vi "log analysis_gps.vi"() -> ()   [LabVIEW 2019] (continued)
 "DUALANTENNAHEADINGA,USB3,0,50.0,FINESTEERING,2107,283656.700,02000000,d426,15824;INSUFFICIENT_OBS,NONE,-1.000000000,0.000000000,0.000000000,0.0,0.000000000,0.000000000,\"631T\",13,4,4,3,04,00,20,03*b691e1de\n\t", "DUALANTENNAHEADINGA,USB3,0,48.0,FINESTEERING,2107,283657.200,02000000,d426,15824;INSUFFICIENT_OBS,NONE,-1.000000000,0.000000000,0.000000000,0.0,0.000000000,0.000000000,\"631T\",13,4,4,3,04,00,20,02*3e465e4d\n\t", "DUALANTENNAHEADINGA,USB3,0,48.0,FINESTEERING,2107,283657.700,02000000,d426,15824;INSUFFICIENT_OBS,NONE,-1.000000000,0.000000000,0.000000000,0.0,0.000000000,0.000000000,\"631T\",13,4,4,3,04,00,20,02*e9554f14\n\t", "INSPVAXA,USB3,0,51.0,FINESTEERING,2107,283658.200,02000000,471d,15824;INS_ALIGNMENT_COMPLETE,INS_RTKFIXED,37.37126197205,126.72203987070,7.8924,22.3000,0.0140,-0.2985,0.0088,-0.407757942,-1.836378522,264.980716512,0.4370,0.2959,0.5779,0.1123,0.0925,0.0785,0.0961,0.1008,5.1265,0f000001,0*c213c735\n\t", "DUALANTENNAHEADINGA,USB3,0,51.0,FINESTEERING,2107,283658.700,02000000,d426,15824;INSUFFICIENT_OBS,NONE,-1.000000000,0.000000000,0.000000000,0.0,0.000000000,0.000000000,\"631T\",14,4,4,3,04,00,20,02*806fba7a\n\t", "DUALANTENNAHEADINGA,USB3,0,45.5,FINESTEERING,2107,283659.200,02000000,d426,15824;INSUFFICIENT_OBS,NONE,-1.000000000,0.000000000,0.000000000,0.0,0.000000000,0.000000000,\"631T\",13,4,4,3,04,00,20,02*be5dbd8b\n\t", "INSPVAXA,USB3,0,45.5,FINESTEERING,2107,283659.700,02000000,471d,15824;INS_ALIGNMENT_COMPLETE,INS_RTKFIXED,37.37126196302,126.72203492233,7.8846,22.3000,0.0219,-0.3038,0.0154,-0.352814130,-1.840091471,265.280226018,0.4363,0.2959,0.5779,0.1123,0.0925,0.0785,0.0961,0.1008,5.1280,0f000001,0*f5025ff3\n\t", "DUALANTENNAHEADINGA,USB3,0,48.5,FINESTEERING,2107,283660.200,02000000,d426,15824;INSUFFICIENT_OBS,NONE,-1.000000000,0.000000000,0.000000000,0.0,0.000000000,0.000000000,\"631T\",14,4,4,3,04,00,20,02*21adfb59\n\t", "DUALANTENNAHEADINGA,USB3,0,48.5,FINESTEERING,2107,283660.700,02000000,d426,15824;INSUFFICIENT_OBS,NONE,-1.000000000,0.000000000,0.000000000,0.0,0.000000000,0.000000000,\"631T\",15,4,4,3,04,00,20,03*565b5ace\n\t", "INSPVAXA,USB3,0,49.5,FINESTEERING,2107,283661.200,02000000,471d,15824;INS_ALIGNMENT_COMPLETE,INS_RTKFIXED,37.37126187130,126.72202999654,7.8827,22.3000,0.0166,-0.2769,0.0144,-0.534535443,-1.728487239,265.001971487,0.4359,0.2961,0.5778,0.1123,0.0926,0.0785,0.0961,0.1008,5.1311,0f000001,0*51cc925f\n\t", "DUALANTENNAHEADINGA,USB3,0,49.5,FINESTEERING,2107,283661.700,02000000,d426,15824;INSUFFICIENT_OBS,NONE,-1.000000000,0.000000000,0.000000000,0.0,0.000000000,0.000000000,\"631T\",12,4,4,3,04,00,20,03*15f903f8\n\t", "DUALANTENNAHEADINGA,USB3,0,48.0,FINESTEERING,2107,283662.200,02000000,d426,15824;INSUFFICIENT_OBS,NONE,-1.000000000,0.000000000,0.000000000,0.0,0.000000000,0.000000000,\"631T\",12,4,4,3,04,00,20,03*45bc2fa2\n\t", "INSPVAXA,USB3,0,48.0,FINESTEERING,2107,283662.700,02000000,471d,15824;INS_ALIGNMENT_COMPLETE,INS_RTKFIXED,37.37126171572,126.72202522799,7.8823,22.3000,-0.0067,-0.2635,0.0136,-1.179961552,0.094212856,265.044425368,0.4362,0.2961,0.5779,0.1131,0.0926,0.0785,0.0961,0.1008,5.1327,0f000001,0*9a1b8d6f\n\t", "DUALANTENNAHEADINGA,USB3,0,49.0,FINESTEERING,2107,283663.200,02000000,d426,15824;INSUFFICIENT_OBS,NONE,-1.000000000,0.000000000,0.000000000,0.0,0.000000000,0.000000000,\"631T\",12,4,4,3,04,00,20,03*4c20fddf\n\t", "DUALANTENNAHEADINGA,USB3,0,49.0,FINESTEERING,2107,283663.700,02000000,d426,15824;INSUFFICIENT_OBS,NONE,-1.000000000,0.000000000,0.000000000,0.0,0.000000000,0.000000000,\"631T\",13,4,4,3,04,00,20,03*4cd16cde\n\t", "DUALANTENNAHEADINGA,USB3,0,53.0,FINESTEERING,2107,283664.200,02000000,d426,15824;INSUFFICIENT_OBS,NONE,-1.000000000,0.000000000,0.000000000,0.0,0.000000000,0.000000000,\"631T\",14,4,4,3,04,00,20,02*f110e9d9\n\t", "DUALANTENNAHEADINGA,USB3,0,53.0,FINESTEERING,2107,283664.700,02000000,d426,15824;INSUFFICIENT_OBS,NONE,-1.000000000,0.000000000,0.000000000,0.0,0.000000000,0.000000000,\"631T\",15,4,4,3,04,00,20,02*f1e178d8\n\t", "DUALANTENNAHEADINGA,USB3,0,50.0,FINESTEERING,2107,283665.200,02000000,d426,15824;INSUFFICIENT_OBS,NONE,-1.000000000,0.000000000,0.000000000,0.0,0.000000000,0.000000000,\"631T\",13,4,4,3,04,00,20,03*0d3c2d31\n\t", "DUALANTENNAHEADINGA,USB3,0,50.0,FINESTEERING,2107,283665.700,02000000,d426,15824;INSUFFICIENT_OBS,NONE,-1.000000000,0.000000000,0.000000000,0.0,0.000000000,0.000000000,\"631T\",12,4,4,3,04,00,20,02*7aca8ca6\n\t", "DUALANTENNAHEADINGA,USB3,0,49.5,FINESTEERING,2107,283666.200,02000000,d426,15824;INSUFFICIENT_OBS,NONE,-1.000000000,0.000000000,0.000000000,0.0,0.000000000,0.000000000,\"631T\",12,4,4,3,04,00,20,03*18930aef\n\t", "DUALANTENNAHEADINGA,USB3,0,51.0,FINESTEERING,2107,283667.200,02000000,d426,15824;INSUFFICIENT_OBS,NONE,-1.000000000,0.000000000,0.000000000,0.0,0.000000000,0.000000000,\"631T\",14,4,4,3,04,00,20,03*f8f6796c\n\t", "DUALANTENNAHEADINGA,USB3,0,51.0,FINESTEERING,2107,283667.700,02000000,d426,15824;INSUFFICIENT_OBS,NONE,-1.000000000,0.000000000,0.000000000,0.0,0.000000000,0.000000000,\"631T\",14,4,4,3,04,00,20,02*58e258a3\n\t", "DUALANTENNAHEADINGA,USB3,0,51.5,FINESTEERING,2107,283668.200,02000000,d426,15824;INSUFFICIENT_OBS,NONE,-1.000000000,0.000000000,0.000000000,0.0,0.000000000,0.000000000,\"631T\",13,4,4,3,04,00,20,03*e5e926ef\n\t", "DUALANTENNAHEADINGA,USB3,0,51.5,FINESTEERING,2107,283668.700,02000000,d426,15824;INSUFFICIENT_OBS,NONE,-1.000000000,0.000000000,0.000000000,0.0,0.000000000,0.000000000,\"631T\",12,4,4,3,04,00,20,03*e518b7ee\n\t", "DUALANTENNAHEADINGA,USB3,0,49.0,FINESTEERING,2107,283669.200,02000000,d426,15824;INSUFFICIENT_OBS,NONE,-1.000000000,0.000000000,0.000000000,0.0,0.000000000,0.000000000,\"631T\",12,4,4,3,04,00,20,03*4fb2de27\n\t", "DUALANTENNAHEADINGA,USB3,0,49.0,FINESTEERING,2107,283669.700,02000000,d426,15824;INSUFFICIENT_OBS,NONE,-1.000000000,0.000000000,0.000000000,0.0,0.000000000,0.000000000,\"631T\",12,4,4,3,04,00,20,02*efa6ffe8\n\t", "DUALANTENNAHEADINGA,USB3,0,50.0,FINESTEERING,2107,283670.200,02000000,d426,15824;INSUFFICIENT_OBS,NONE,-1.000000000,0.000000000,0.000000000,0.0,0.000000000,0.000000000,\"631T\",12,4,4,3,04,00,20,03*24750ee1\n\t", "DUALANTENNAHEADINGA,USB3,0,50.0,FINESTEERING,2107,283670.700,02000000,d426,15824;INSUFFICIENT_OBS,NONE,-1.000000000,0.000000000,0.000000000,0.0,0.000000000,0.000000000,\"631T\",13,4,4,3,04,00,20,03*24849fe0\n\t", "DUALANTENNAHEADINGA,USB3,0,50.0,FINESTEERING,2107,283671.200,02000000,d426,15824;INSUFFICIENT_OBS,NONE,-1.000000000,0.000000000,0.000000000,0.0,0.000000000,0.000000000,\"631T\",13,4,4,3,04,00,20,02*e948baf6\n\t", "DUALANTENNAHEADINGA,USB3,0,50.0,FINESTEERING,2107,283671.700,02000000,d426,15824;INSUFFICIENT_OBS,NONE,-1.000000000,0.000000000,0.000000000,0.0,0.000000000,0.000000000,\"631T\",12,4,4,3,04,00,20,02*e9b92bf7\n\t", "DUALANTENNAHEADINGA,USB3,0,47.5,FINESTEERING,2107,283672.200,02000000,d426,15824;INSUFFICIENT_OBS,NONE,-1.000000000,0.000000000,0.000000000,0.0,0.000000000,0.000000000,\"631T\",13,4,4,3,04,00,20,03*4a2d65dd\n\t", "DUALANTENNAHEADINGA,USB3,0,47.5,FINESTEERING,2107,283672.700,02000000,d426,15824;INSUFFICIENT_OBS,NONE,-1.000000000,0.000000000,0.000000000,0.0,0.000000000,0.000000000,\"631T\",11,4,4,3,04,00,20,03*e98a7275\n\t", "DUALANTENNAHEADINGA,USB3,0,49.0,FINESTEERING,2107,283673.200,02000000,d426,15824;INSUFFICIENT_OBS,NONE,-1.000000000,0.000000000,0.000000000,0.0,0.000000000,0.000000000,\"631T\",12,4,4,3,04,00,20,02*c4457f3d\n\t", "DUALANTENNAHEADINGA,USB3,0,49.0,FINESTEERING,2107,283673.700,02000000,d426,15824;INSUFFICIENT_OBS,NONE,-1.000000000,0.000000000,0.000000000,0.0,0.000000000,0.000000000,\"631T\",13,4,4,3,04,00,20,03*b3b3deaa\n\t", "DUALANTENNAHEADINGA,USB3,0,50.0,FINESTEERING,2107,283674.200,02000000,d426,15824;INSUFFICIENT_OBS,NONE,-1.000000000,0.000000000,0.000000000,0.0,0.000000000,0.000000000,\"631T\",13,4,4,3,04,00,20,03*9f869b9c\n\t", "INSPVAXA,USB3,0,50.0,FINESTEERING,2107,283674.750,02000000,471d,15824;INS_ALIGNMENT_COMPLETE,INS_RTKFIXED,37.37126252882,126.72198672229,7.9795,22.3000,-0.0186,-0.2998,0.0327,-1.236759140,0.298585225,263.242315357,0.4398,0.2975,0.5789,0.1131,0.0929,0.0786,0.0960,0.1008,5.0828,0f000001,0*30bc741b\n\t", "DUALANTENNAHEADINGA,USB3,0,47.5,FINESTEERING,2107,283675.200,02000000,d426,15824;INSUFFICIENT_OBS,NONE,-1.000000000,0.000000000,0.000000000,0.0,0.000000000,0.000000000,\"631T\",12,4,4,3,04,00,20,02*30b1cd5d\n\t", "DUALANTENNAHEADINGA,USB3,0,47.5,FINESTEERING,2107,283675.700,02000000,d426,15824;INSUFFICIENT_OBS,NONE,-1.000000000,0.000000000,0.000000000,0.0,0.000000000,0.000000000,\"631T\",13,4,4,3,04,00,20,03*47476cca\n\t", "DUALANTENNAHEADINGA,USB3,0,50.0,FINESTEERING,2107,283676.200,02000000,d426,15824;INSUFFICIENT_OBS,NONE,-1.000000000,0.000000000,0.000000000,0.0,0.000000000,0.000000000,\"631T\",13,4,4,3,04,00,20,02*3331a2b8\n\t", "INSPVAXA,USB3,0,50.0,FINESTEERING,2107,283676.750,02000000,471d,15824;INS_ALIGNMENT_COMPLETE,INS_RTKFIXED,37.37126202802,126.72198037867,7.9931,22.3000,-0.0270,-0.2983,0.0289,-1.276938431,0.174085147,258.154591337,0.4371,0.2976,0.5788,0.1128,0.0927,0.0785,0.0959,0.1007,5.0828,0f000001,0*1eb9a34f\n\t", "INSPVAXA,USB3,0,47.5,FINESTEERING,2107,283677.250,02000000,471d,15824;INS_ALIGNMENT_COMPLETE,INS_RTKFIXED,37.37126184306,126.72197878066,7.9954,22.3000,-0.0249,-0.2800,0.0095,-1.329008924,0.068233484,257.455385518,0.4363,0.2976,0.5789,0.1128,0.0926,0.0785,0.0959,0.1006,5.0823,0f000001,0*a0488656\n\t", "INSPVAXA,USB3,0,44.5,FINESTEERING,2107,283678.750,02000000,471d,15824;INS_ALIGNMENT_COMPLETE,INS_RTKFIXED,37.37126126052,126.72197417876,8.0025,22.3000,-0.0388,-0.3139,0.0075,-1.341441151,0.143163163,255.994609032,0.4352,0.2975,0.5790,0.1123,0.0928,0.0785,0.0959,0.1006,5.0816,0f000001,0*2dcb75ae\n\t", "INSPVAXA,USB3,0,50.0,FINESTEERING,2107,283679.250,02000000,471d,15824;INS_ALIGNMENT_COMPLETE,INS_RTKFIXED,37.37126102386,126.72197256335,8.0029,22.3000,-0.0378,-0.3051,0.0239,-1.252291621,0.317106039,255.710782643,0.4355,0.2977,0.5792,0.1125,0.0927,0.0786,0.0959,0.1006,5.0819,0f000001,0*497f861f\n\t", "DUALANTENNAHEADINGA,USB3,0,50.0,FINESTEERING,2107,283679.700,02000000,d426,15824;INSUFFICIENT_OBS,NONE,-1.000000000,0.000000000,0.000000000,0.0,0.000000000,0.000000000,\"631T\",13,4,4,3,04,00,20,03*917eb173\n\t", "INSPVAXA,USB3,0,49.5,FINESTEERING,2107,283680.250,02000000,471d,15824;INS_ALIGNMENT_COMPLETE,INS_RTKFIXED,37.37126052998,126.72196935056,8.0055,22.3000,-0.0369,-0.2979,0.0271,-1.221523222,0.248269535,255.390291305,0.4350,0.2975,0.5791,0.1126,0.0927,0.0786,0.0959,0.1006,5.0824,0f000001,0*4c9222e8\n\t", "INSPVAXA,USB3,0,49.5,FINESTEERING,2107,283680.750,02000000,471d,15824;INS_ALIGNMENT_COMPLETE,INS_RTKFIXED,37.37126029067,126.72196774054,8.0075,22.3000,-0.0484,-0.2930,0.0156,-1.123777574,0.215686141,255.306454627,0.4350,0.2975,0.5791,0.1126,0.0927,0.0786,0.0959,0.1006,5.0824,0f000001,0*b1d08eab\n\t", "DUALANTENNAHEADINGA,USB3,0,47.5,FINESTEERING,2107,283681.200,02000000,d426,15824;INSUFFICIENT_OBS,NONE,-1.000000000,0.000000000,0.000000000,0.0,0.000000000,0.000000000,\"631T\",13,4,4,3,04,00,20,02*8c2dc70b\n\t", "DUALANTENNAHEADINGA,USB3,0,47.5,FINESTEERING,2107,283681.700,02000000,d426,15824;INSUFFICIENT_OBS,NONE,-1.000000000,0.000000000,0.000000000,0.0,0.000000000,0.000000000,\"631T\",13,4,4,3,04,00,20,03*2c39e6c4\n\t", "DUALANTENNAHEADINGA,USB3,0,53.0,FINESTEERING,2107,283682.200,02000000,d426,15824;INSUFFICIENT_OBS,NONE,-1.000000000,0.000000000,0.000000000,0.0,0.000000000,0.000000000,\"631T\",13,4,4,3,04,00,20,02*f482535a\n\t", "INSPVAXA,USB3,0,53.0,FINESTEERING,2107,283682.750,02000000,471d,15824;INS_ALIGNMENT_COMPLETE,INS_RTKFIXED,37.37125926494,126.72196137618,8.0142,22.3000,-0.0531,-0.2940,0.0193,-1.467222683,0.192661373,255.088191975,0.4346,0.2973,0.5792,0.1126,0.0928,0.0786,0.0959,0.1005,5.0834,0f000001,0*e49cbeff\n\t", "DUALANTENNAHEADINGA,USB3,0,51.5,FINESTEERING,2107,283683.200,02000000,d426,15824;INSUFFICIENT_OBS,NONE,-1.000000000,0.000000000,0.000000000,0.0,0.000000000,0.000000000,\"631T\",13,4,4,3,04,00,20,03*73ae2c91\n\t", "INSPVAXA,USB3,0,51.5,FINESTEERING,2107,283683.750,02000000,471d,15824;INS_ALIGNMENT_COMPLETE,INS_RTKFIXED,37.37125874592,126.72195815928,8.0147,22.3000,-0.0440,-0.2967,0.0132,-1.341050050,-0.067435832,254.924614252,0.4345,0.2971,0.5791,0.1126,0.0928,0.0785,0.0959,0.1005,5.0840,0f000001,0*701f89f0\n\t", "DUALANTENNAHEADINGA,USB3,0,52.0,FINESTEERING,2107,283684.200,02000000,d426,15824;INSUFFICIENT_OBS,NONE,-1.000000000,0.000000000,0.000000000,0.0,0.000000000,0.000000000,\"631T\",13,4,4,3,04,00,20,02*27679969\n\t", "INSPVAXA,USB3,0,52.0,FINESTEERING,2107,283684.750,02000000,471d,15824;INS_ALIGNMENT_COMPLETE,INS_RTKFIXED,37.37125823226,126.72195499542,8.0159,22.3000,-0.0425,-0.2912,0.0233,-1.481512417,-0.232627459,254.717814630,0.4345,0.2970,0.5790,0.1126,0.0928,0.0785,0.0959,0.1005,5.0847,0f000001,0*bc004070\n\t", "DUALANTENNAHEADINGA,USB3,0,54.0,FINESTEERING,2107,283685.200,02000000,d426,15824;INSUFFICIENT_OBS,NONE,-1.000000000,0.000000000,0.000000000,0.0,0.000000000,0.000000000,\"631T\",13,4,4,3,04,00,20,03*bf535cbf\n\t", "DUALANTENNAHEADINGA,USB3,0,54.0,FINESTEERING,2107,283685.700,02000000,d426,15824;INSUFFICIENT_OBS,NONE,-1.000000000,0.000000000,0.000000000,0.0,0.000000000,0.000000000,\"631T\",15,4,4,3,04,00,20,03*f59c46f5\n\t", "INSPVAXA,USB3,0,47.0,FINESTEERING,2107,283686.250,02000000,471d,15824;INS_ALIGNMENT_COMPLETE,INS_RTKFIXED,37.37125745168,126.72195028422,8.0177,22.3000,-0.0421,-0.2788,0.0295,-1.327379585,-0.197998940,254.015433265,0.4342,0.2970,0.5788,0.1125,0.0928,0.0785,0.0959,0.1004,5.0859,0f000001,0*059a606c\n\t", "INSPVAXA,USB3,0,47.0,FINESTEERING,2107,283686.750,02000000,471d,15824;INS_ALIGNMENT_COMPLETE,INS_RTKFIXED,37.37125719652,126.72194873669,8.0201,22.3000,-0.0424,-0.2865,0.0311,-1.155721868,-0.143426026,253.623399398,0.4342,0.2970,0.5788,0.1125,0.0928,0.0785,0.0959,0.1004,5.0859,0f000001,0*874a06ff\n\t", "INSPVAXA,USB3,0,48.5,FINESTEERING,2107,283687.250,02000000,471d,15824;INS_ALIGNMENT_COMPLETE,INS_RTKFIXED,37.37125692308,126.72194717786,8.0216,22.3000,-0.0335,-0.2418,0.0315,-1.192319582,-0.154191109,253.231237079,0.4341,0.2971,0.5788,0.1124,0.0928,0.0785,0.0959,0.1004,5.0866,0f000001,0*54818d56\n\t", "INSPVAXA,USB3,0,48.0,FINESTEERING,2107,283688.250,02000000,471d,15824;INS_ALIGNMENT_COMPLETE,INS_RTKFIXED,37.37125642172,126.72194437677,8.0235,22.3000,-0.0500,-0.3046,0.0059,-1.164662178,-0.014385646,252.588332690,0.4343,0.2973,0.5789,0.1124,0.0928,0.0785,0.0959,0.1004,5.0876,0f000001,0*78a62f40\n\t", "INSPVAXA,USB3,0,48.0,FINESTEERING,2107,283688.750,02000000,471d,15824;INS_ALIGNMENT_COMPLETE,INS_RTKFIXED,37.37125610282,126.72194283979,8.0244,22.3000,-0.0543,-0.2923,0.0224,-1.111219856,-0.008949492,252.070206998,0.4343,0.2973,0.5789,0.1124,0.0928,0.0785,0.0959,0.1004,5.0876,0f000001,0*c44a5f5d\n\t", "INSPVAXA,USB3,0,50.0,FINESTEERING,2107,283689.250,02000000,471d,15824;INS_ALIGNMENT_COMPLETE,INS_RTKFIXED,37.37125577091,126.72194129043,8.0250,22.3000,-0.0553,-0.2846,0.0299,-1.126484070,-0.034453614,251.571777713,0.4347,0.2976,0.5789,0.1123,0.0927,0.0785,0.0959,0.1004,5.0890,0f000001,0*4752c184\n\t", "INSPVAXA,USB3,0,50.0,FINESTEERING,2107,283689.750,02000000,471d,15824;INS_ALIGNMENT_COMPLETE,INS_RTKFIXED,37.37125543079,126.72193970784,8.0254,22.3000,-0.0623,-0.2845,0.0344,-1.115085970,-0.181471482,251.113733002,0.4347,0.2976,0.5789,0.1123,0.0927,0.0785,0.0959,0.1004,5.0890,0f000001,0*e6043553\n\t", "INSPVAXA,USB3,0,51.5,FINESTEERING,2107,283690.250,02000000,471d,15824;INS_ALIGNMENT_COMPLETE,INS_RTKFIXED,37.37125508435,126.72193816260,8.0268,22.3000,-0.0829,-0.2745,0.0314,-1.131096634,-0.362526816,250.672431743,0.4348,0.2977,0.5789,0.1123,0.0927,0.0785,0.0959,0.1004,5.0905,0f000001,0*0f3c6f4d\n\t", "INSPVAXA,USB3,0,51.5,FINESTEERING,2107,283690.750,02000000,471d,15824;INS_ALIGNMENT_COMPLETE,INS_RTKFIXED,37.37125472381,126.72193660268,8.0270,22.3000,-0.0761,-0.2693,0.0189,-1.124428932,-0.555258111,250.148936400,0.4348,0.2977,0.5789,0.1123,0.0927,0.0785,0.0959,0.1004,5.0905,0f000001,0*bccc2e0c\n\t", "INSPVAXA,USB3,0,51.0,FINESTEERING,2107,283691.250,02000000,471d,15824;INS_ALIGNMENT_COMPLETE,INS_RTKFIXED,37.37125435874,126.72193505456,8.0263,22.3000,-0.0670,-0.2696,0.0092,-1.064456242,-0.547416950,249.737681282,0.4347,0.2977,0.5789,0.1123,0.0927,0.0785,0.0959,0.1004,5.0921,0f000001,0*f2a7f55d\n\t", "INSPVAXA,USB3,0,51.0,FINESTEERING,2107,283691.750,02000000,471d,15824;INS_ALIGNMENT_COMPLETE,INS_RTKFIXED,37.37125397017,126.72193349362,8.0255,22.3000,-0.0691,-0.2936,0.0158,-1.034003666,-0.605283129,249.246949956,0.4347,0.2977,0.5789,0.1123,0.0927,0.0785,0.0959,0.1004,5.0921,0f000001,0*27b79f83\n\t", "INSPVAXA,USB3,0,52.0,FINESTEERING,2107,283692.250,02000000,471d,15824;INS_ALIGNMENT_COMPLETE,INS_RTKFIXED,37.37125358988,126.72193199872,8.0234,22.3000,-0.0664,-0.2884,0.0105,-1.029506848,-0.448748893,248.703805210,0.4344,0.2976,0.5789,0.1123,0.0927,0.0785,0.0960,0.1004,5.0936,0f000001,0*b0abd4b9\n\t", "INSPVAXA,USB3,0,52.0,FINESTEERING,2107,283692.750,02000000,471d,15824;INS_ALIGNMENT_COMPLETE,INS_RTKFIXED,37.37125319556,126.72193048668,8.0218,22.3000,-0.0721,-0.2829,0.0182,-0.873709041,-0.554913446,248.258505340,0.4344,0.2976,0.5789,0.1123,0.0927,0.0785,0.0960,0.1004,5.0936,0f000001,0*33541c24\n\t", "INSPVAXA,USB3,0,52.0,FINESTEERING,2107,283693.250,02000000,471d,15824;INS_ALIGNMENT_COMPLETE,INS_RTKFIXED,37.37125278430,126.72192895782,8.0198,22.3000,-0.0808,-0.2833,0.0124,-0.750595920,-0.512604817,247.887825209,0.4345,0.2977,0.5790,0.1123,0.0927,0.0785,0.0960,0.1005,5.0951,0f000001,0*33503232\n\t", "INSPVAXA,USB3,0,52.0,FINESTEERING,2107,283693.750,02000000,471d,15824;INS_ALIGNMENT_COMPLETE,INS_RTKFIXED,37.37125237385,126.72192745643,8.0181,22.3000,-0.0699,-0.2766,0.0107,-0.708441706,-0.569028922,247.469165126,0.4345,0.2977,0.5790,0.1123,0.0927,0.0785,0.0960,0.1005,5.0951,0f000001,0*b12f53f8\n\t", "INSPVAXA,USB3,0,51.5,FINESTEERING,2107,283694.250,02000000,471d,15824;INS_ALIGNMENT_COMPLETE,INS_RTKFIXED,37.37125195619,126.72192597903,8.0151,22.3000,-0.0814,-0.2811,0.0110,-0.711365496,-0.463120250,247.118464084,0.4343,0.2979,0.5790,0.1123,0.0927,0.0785,0.0960,0.1005,5.0966,0f000001,0*fc596ab1\n\t", "INSPVAXA,USB3,0,51.5,FINESTEERING,2107,283694.750,02000000,471d,15824;INS_ALIGNMENT_COMPLETE,INS_RTKFIXED,37.37125151893,126.72192448231,8.0119,22.3000,-0.0800,-0.2663,0.0091,-0.771660159,-0.376939407,246.768281160,0.4343,0.2979,0.5790,0.1123,0.0927,0.0785,0.0960,0.1005,5.0966,0f000001,0*6d22b1be\n\t", "INSPVAXA,USB3,0,48.0,FINESTEERING,2107,283695.250,02000000,471d,15824;INS_ALIGNMENT_COMPLETE,INS_RTKFIXED,37.37125106123,126.72192297885,8.0100,22.3000,-0.0761,-0.2505,0.0231,-0.897100380,-0.291610583,246.370264659,0.4345,0.2982,0.5790,0.1123,0.0927,0.0785,0.0960,0.1005,5.0981,0f000001,0*3984aa9f\n\t", "INSPVAXA,USB3,0,48.0,FINESTEERING,2107,283695.750,02000000,471d,15824;INS_ALIGNMENT_COMPLETE,INS_RTKFIXED,37.37125059397,126.72192150260,8.0095,22.3000,-0.0806,-0.2555,0.0180,-1.082975458,-0.280956917,246.024954508,0.4345,0.2982,0.5790,0.1123,0.0927,0.0785,0.0960,0.1005,5.0981,0f000001,0*61086754\n\t", "INSPVAXA,USB3,0,48.5,FINESTEERING,2107,283696.250,02000000,471d,15824;INS_ALIGNMENT_COMPLETE,INS_RTKFIXED,37.37125013310,126.72192002149,8.0081,22.3000,-0.0880,-0.2655,0.0330,-1.084281837,-0.279647129,245.685810619,0.4346,0.2982,0.5792,0.1123,0.0927,0.0785,0.0960,0.1005,5.0996,0f000001,0*ddc3e251\n\t", "INSPVAXA,USB3,0,48.5,FINESTEERING,2107,283696.750,02000000,471d,15824;INS_ALIGNMENT_COMPLETE,INS_RTKFIXED,37.37124978634,126.72191884253,8.0066,22.3000,0.0400,0.0236,0.0167,-1.049670935,-0.308268923,245.402478860,0.4346,0.2982,0.5792,0.1123,0.0927,0.0785,0.0960,0.1005,5.0996,0f000001,0*5343d95d\n\t", "INSPVAXA,USB3,0,49.5,FINESTEERING,2107,283697.250,02000000,471d,15824;INS_ALIGNMENT_COMPLETE,INS_RTKFIXED,37.37124936191,126.72191751580,8.0075,22.3000,-0.0790,-0.2224,0.0305,-1.160332211,-0.255386119,245.257033584,0.4348,0.2981,0.5792,0.1123,0.0927,0.0785,0.0960,0.1005,5.1012,0f000001,0*9bb241a9\n\t", "INSPVAXA,USB3,0,49.5,FINESTEERING,2107,283697.750,02000000,471d,15824;INS_ALIGNMENT_COMPLETE,INS_RTKFIXED,37.37124887882,126.72191610954,8.0072,22.3000,-0.0796,-0.2609,0.0250,-1.450872911,-0.189081024,245.072886035,0.4348,0.2981,0.5792,0.1123,0.0927,0.0785,0.0960,0.1005,5.1012,0f000001,0*ca3e42a8\n\t", "INSPVAXA,USB3,0,47.0,FINESTEERING,2107,283698.250,02000000,471d,15824;INS_ALIGNMENT_COMPLETE,INS_RTKFIXED,37.37124839401,126.72191465708,8.0076,22.3000,-0.0773,-0.2590,0.0230,-1.479636169,-0.110505972,244.843169403,0.4347,0.2979,0.5791,0.1126,0.0927,0.0785,0.0960,0.1005,5.1027,0f000001,0*0006d84b\n\t", "INSPVAXA,USB3,0,47.0,FINESTEERING,2107,283698.750,02000000,471d,15824;INS_ALIGNMENT_COMPLETE,INS_RTKFIXED,37.37124790607,126.72191317649,8.0096,22.3000,-0.0919,-0.2605,0.0162,-1.323665543,0.178775756,244.574454938,0.4347,0.2979,0.5791,0.1126,0.0927,0.0785,0.0960,0.1005,5.1027,0f000001,0*97fdd670\n\t", "INSPVAXA,USB3,0,47.5,FINESTEERING,2107,283699.250,02000000,471d,15824;INS_ALIGNMENT_COMPLETE,INS_RTKFIXED,37.37124741280,126.72191168515,8.0116,22.3000,-0.0880,-0.2650,0.0236,-1.277654114,0.173050319,244.335495990,0.4352,0.2978,0.5791,0.1127,0.0927,0.0785,0.0959,0.1005,5.1036,0f000001,0*401d1919\n\t", "INSPVAXA,USB3,0,47.5,FINESTEERING,2107,283699.750,02000000,471d,15824;INS_ALIGNMENT_COMPLETE,INS_RTKFIXED,37.37124691977,126.72191021065,8.0139,22.3000,-0.0941,-0.2573,0.0260,-1.295740084,0.118148751,244.043765881,0.4352,0.2978,0.5791,0.1127,0.0927,0.0785,0.0959,0.1005,5.1036,0f000001,0*b4e001ab\n\t", "INSPVAXA,USB3,0,48.5,FINESTEERING,2107,283700.250,02000000,471d,15824;INS_ALIGNMENT_COMPLETE,INS_RTKFIXED,37.37124641299,126.72190870241,8.0157,22.3000,-0.0965,-0.2606,0.0330,-1.289006516,0.186517966,243.733079989,0.4358,0.2981,0.5791,0.1128,0.0927,0.0785,0.0959,0.1005,5.1040,0f000001,0*7b588f65\n\t", "INSPVAXA,USB3,0,48.5,FINESTEERING,2107,283700.750,02000000,471d,15824;INS_ALIGNMENT_COMPLETE,INS_RTKFIXED,37.37124591211,126.72190719117,8.0183,22.3000,-0.0934,-0.2790,0.0272,-1.230862677,0.124809038,243.414753616,0.4358,0.2981,0.5791,0.1128,0.0927,0.0785,0.0959,0.1005,5.1040,0f000001,0*24944499\n\t", "INSPVAXA,USB3,0,48.0,FINESTEERING,2107,283701.250,02000000,471d,15824;INS_ALIGNMENT_COMPLETE,INS_RTKFIXED,37.37124542632,126.72190568049,8.0217,22.3000,-0.0782,-0.2571,0.0284,-0.983799928,0.018605262,242.857861412,0.4361,0.2983,0.5790,0.1125,0.0928,0.0785,0.0959,0.1004,5.1037,0f000001,0*579729be\n\t", "INSPVAXA,USB3,0,48.0,FINESTEERING,2107,283701.750,02000000,471d,15824;INS_ALIGNMENT_COMPLETE,INS_RTKFIXED,37.37124504941,126.72190455554,8.0252,22.3000,-0.1066,-0.3087,0.0271,-0.874891899,0.189008715,240.527059520,0.4361,0.2983,0.5790,0.1125,0.0928,0.0785,0.0959,0.1004,5.1037,0f000001,0*9bbd18ba\n\t", "INSPVAXA,USB3,0,50.5,FINESTEERING,2107,283702.250,02008000,471d,15824;INS_ALIGNMENT_COMPLETE,INS_RTKFIXED,37.37124442762,126.72190307020,8.0282,22.3000,-0.1382,-0.2404,0.0216,-0.866741092,0.060143860,235.368916733,0.4360,0.2989,0.5791,0.1125,0.0927,0.0785,0.0959,0.1004,5.1028,0f000001,0*0ab995b1\n\t", "INSPVAXA,USB3,0,50.5,FINESTEERING,2107,283702.750,02008000,471d,15824;INS_ALIGNMENT_COMPLETE,INS_RTKFIXED,37.37124370430,126.72190170598,8.0314,22.3000,-0.1609,-0.2382,0.0230,-1.064164970,-0.109212362,230.360783935,0.4360,0.2989,0.5791,0.1125,0.0927,0.0785,0.0959,0.1004,5.1028,0f000001,0*391c17ea\n\t", "INSPVAXA,USB3,0,50.5,FINESTEERING,2107,283703.250,02008000,471d,15824;INS_ALIGNMENT_COMPLETE,INS_RTKFIXED,37.37124291299,126.72190041379,8.0333,22.3000,-0.1952,-0.2293,0.0238,-0.984755093,-0.132867348,225.970025862,0.4356,0.2991,0.5791,0.1126,0.0928,0.0785,0.0959,0.1003,5.0999,0f000001,0*698b4567\n\t", "INSPVAXA,USB3,0,50.5,FINESTEERING,2107,283703.750,02008000,471d,15824;INS_ALIGNMENT_COMPLETE,INS_RTKFIXED,37.37124204915,126.72189921350,8.0352,22.3000,-0.1844,-0.2111,0.0260,-0.917701758,-0.201673518,222.401686882,0.4356,0.2991,0.5791,0.1126,0.0928,0.0785,0.0959,0.1003,5.0999,0f000001,0*b00298a2\n\t", "INSPVAXA,USB3,0,52.5,FINESTEERING,2107,283704.250,02008000,471d,15824;INS_ALIGNMENT_COMPLETE,INS_RTKFIXED,37.37124115069,126.72189807141,8.0376,22.3000,-0.2004,-0.2048,0.0174,-1.022423432,-0.388489047,219.876868420,0.4350,0.2996,0.5792,0.1127,0.0932,0.0785,0.0959,0.1002,5.0962,0f000001,0*a3ed39a7\n\t", "INSPVAXA,USB3,0,49.0,FINESTEERING,2107,283706.250,02000000,471d,15824;INS_ALIGNMENT_COMPLETE,INS_RTKFIXED,37.37123727449,126.72189373290,8.0459,22.3000,-0.2128,-0.1725,0.0234,-1.209481692,-0.641915990,215.491722437,0.4342,0.2996,0.5792,0.1131,0.0940,0.0785,0.0958,0.1000,5.0896,0f000001,0*17f33bf8\n\t", "INSPVAXA,USB3,0,48.0,FINESTEERING,2107,283708.750,02000000,471d,15824;INS_ALIGNMENT_COMPLETE,INS_RTKFIXED,37.37123243346,126.72188856798,8.0524,22.3000,-0.2261,-0.1988,0.0348,-0.901144389,0.198517088,216.068250982,0.4339,0.3000,0.5792,0.1135,0.0940,0.0785,0.0956,0.0997,5.0860,0f000001,0*ba7ccbe0\n\t", "INSPVAXA,USB3,0,47.5,FINESTEERING,2107,283709.250,02000000,471d,15824;INS_ALIGNMENT_COMPLETE,INS_RTKFIXED,37.37123135236,126.72188744771,8.0521,22.3000,-0.2176,-0.2013,0.0343,-0.897424345,0.439323734,216.334218434,0.4339,0.3008,0.5792,0.1136,0.0941,0.0785,0.0955,0.0996,5.0867,0f000001,0*2487740e\n\t", "INSPVAXA,USB3,0,46.5,FINESTEERING,2107,283711.750,02000000,471d,15824;INS_ALIGNMENT_COMPLETE,INS_RTKFIXED,37.37122661325,126.72188206330,8.0523,22.3000,-0.1946,-0.1990,0.0081,-0.343732019,-0.465256456,221.217414786,0.4342,0.3030,0.5793,0.1138,0.0937,0.0785,0.0954,0.0993,5.0883,0f000001,0*d2ab07a9\n\t", "INSPVAXA,USB3,0,44.5,FINESTEERING,2107,283712.250,02000000,471d,15824;INS_ALIGNMENT_COMPLETE,INS_RTKFIXED,37.37122571809,126.72188087797,8.0513,22.3000,-0.1877,-0.2276,0.0316,0.179753839,-0.491470448,222.605830014,0.4342,0.3024,0.5794,0.1134,0.0940,0.0785,0.0954,0.0992,5.0887,0f000001,0*82158439\n\t", "INSPVAXA,USB3,0,49.5,FINESTEERING,2107,283715.750,02000000,471d,15824;INS_ALIGNMENT_COMPLETE,INS_RTKFIXED,37.37122004093,126.72187255202,8.0310,22.3000,-0.2525,-0.3284,0.0150,-0.722312377,-0.111566034,228.459144624,0.4339,0.3022,0.5793,0.1124,0.0928,0.0785,0.0954,0.0992,5.0842,0f000001,0*1d534d62\n\t", "INSPVAXA,USB3,0,50.0,FINESTEERING,2107,283731.800,02000000,471d,15824;INS_ALIGNMENT_COMPLETE,INS_RTKFIXED,37.37117458679,126.72181307353,7.9818,22.3000,-0.3273,-0.2857,0.0109,-1.190065034,-0.069687290,213.721334289,0.4352,0.3028,0.5840,0.1128,0.0931,0.0809,0.0959,0.1000,5.0570,0f000001,0*9dfc8b18\n\t", "INSPVAXA,USB3,0,51.0,FINESTEERING,2107,283732.800,02000000,471d,15824;INS_ALIGNMENT_COMPLETE,INS_RTKFIXED,37.37117121797,126.72180974634,7.9878,22.3000,-0.3313,-0.2857,0.0219,-1.270635454,-0.215524516,213.339771314,0.4352,0.3028,0.5846,0.1129,0.0933,0.0811,0.0960,0.1001,5.0551,0f000001,0*0aee9a35\n\t", "INSPVAXA,USB3,0,51.5,FINESTEERING,2107,283733.300,02000000,471d,15824;INS_ALIGNMENT_COMPLETE,INS_RTKFIXED,37.37116954427,126.72180813326,7.9908,22.3000,-0.3552,-0.2859,0.0156,-1.448481440,-0.233169639,213.103409582,0.4350,0.3026,0.5849,0.1127,0.0932,0.0807,0.0961,0.1001,5.0540,0f000001,0*6eded770\n\t", "INSPVAXA,USB3,0,50.5,FINESTEERING,2107,283734.300,02000000,471d,15824;INS_ALIGNMENT_COMPLETE,INS_RTKFIXED,37.37116643278,126.72180513242,7.9941,22.3000,-0.3478,-0.2920,-0.0081,-1.453049667,-0.445591431,212.491210472,0.4347,0.3023,0.5850,0.1126,0.0932,0.0804,0.0961,0.1001,5.0539,0f000001,0*79c2ad3a\n\t", "INSPVAXA,USB3,0,50.0,FINESTEERING,2107,283735.800,02000000,471d,15824;INS_ALIGNMENT_COMPLETE,INS_RTKFIXED,37.37116119506,126.72180032977,8.0024,22.3000,-0.3542,-0.2959,0.0116,-1.070253035,-0.077101790,211.926024212,0.4346,0.3023,0.5850,0.1127,0.0933,0.0801,0.0962,0.1001,5.0543,0f000001,0*c680b455\n\t", "INSPVAXA,USB3,0,52.5,FINESTEERING,2107,283736.300,02000000,471d,15824;INS_ALIGNMENT_COMPLETE,INS_RTKFIXED,37.37115947932,126.72179880714,8.0040,22.3000,-0.3644,-0.2930,0.0272,-1.158322238,-0.026079764,211.769815237,0.4340,0.3014,0.5849,0.1129,0.0936,0.0802,0.0962,0.1001,5.0557,0f000001,0*91878766\n\t", "INSPVAXA,USB3,0,49.5,FINESTEERING,2107,283737.300,02000000,471d,15824;INS_ALIGNMENT_COMPLETE,INS_RTKFIXED,37.37115601705,126.72179575213,8.0111,22.3000,-0.3535,-0.2715,0.0236,-1.072991275,-0.157444358,211.337264747,0.4338,0.3020,0.5848,0.1128,0.0935,0.0799,0.0962,0.1000,5.0571,0f000001,0*fcfec35c\n\t", "INSPVAXA,USB3,0,49.5,FINESTEERING,2107,283737.800,02000000,471d,15824;INS_ALIGNMENT_COMPLETE,INS_RTKFIXED,37.37115424403,126.72179422575,8.0146,22.3000,-0.3686,-0.2725,0.0313,-1.104138059,-0.177331016,211.359293731,0.4338,0.3020,0.5848,0.1128,0.0935,0.0799,0.0962,0.1000,5.0571,0f000001,0*ab5647ea\n\t", "INSPVAXA,USB3,0,49.5,FINESTEERING,2107,283739.300,02000000,471d,15824;INS_ALIGNMENT_COMPLETE,INS_RTKFIXED,37.37114934907,126.72178999234,8.0211,22.3000,-0.4739,-0.3464,0.0176,-1.136581936,-0.167253224,210.967892029,0.4333,0.3019,0.5842,0.1128,0.0941,0.0795,0.0961,0.1000,5.0600,0f000001,0*70943433\n\t", "INSPVAXA,USB3,0,50.0,FINESTEERING,2107,283740.800,02000000,471d,15824;INS_ALIGNMENT_COMPLETE,INS_RTKFIXED,37.37114414583,126.72178561946,8.0225,22.3000,-0.3822,-0.2779,0.0042,-1.093019003,-0.010151528,210.947598498,0.4332,0.3033,0.5839,0.1127,0.0932,0.0793,0.0961,0.0999,5.0603,0f000001,0*1136f991\n\t", "INSPVAXA,USB3,0,48.5,FINESTEERING,2107,283741.800,02000000,471d,15824;INS_ALIGNMENT_COMPLETE,INS_RTKFIXED,37.37114058594,126.72178265531,8.0253,22.3000,-0.3567,-0.2593,0.0215,-1.513936100,-0.057286463,211.372668569,0.4332,0.3024,0.5836,0.1132,0.0938,0.0801,0.0960,0.0999,5.0615,0f000001,0*2f761fac\n\t", "INSPVAXA,USB3,0,48.5,FINESTEERING,2107,283742.300,02000000,471d,15824;INS_ALIGNMENT_COMPLETE,INS_RTKFIXED,37.37113883610,126.72178116483,8.0251,22.3000,-0.3566,-0.2646,-0.0002,-1.629553261,-0.371874785,211.544863069,0.4334,0.3022,0.5834,0.1130,0.0935,0.0799,0.0960,0.0999,5.0629,0f000001,0*db798f34\n\t", "INSPVAXA,USB3,0,48.5,FINESTEERING,2107,283742.800,02000000,471d,15824;INS_ALIGNMENT_COMPLETE,INS_RTKFIXED,37.37113713184,126.72177968059,8.0243,22.3000,-0.3489,-0.2579,0.0216,-1.473854332,-0.365287327,211.722184950,0.4334,0.3022,0.5834,0.1130,0.0935,0.0799,0.0960,0.0999,5.0629,0f000001,0*7daa81b7\n\t", "INSPVAXA,USB3,0,46.0,FINESTEERING,2107,283743.300,02000000,471d,15824;INS_ALIGNMENT_COMPLETE,INS_RTKFIXED,37.37113541318,126.72177817924,8.0241,22.3000,-0.3602,-0.2594,0.0280,-1.547897785,-0.197369444,211.857866163,0.4337,0.3019,0.5833,0.1132,0.0937,0.0803,0.0960,0.0999,5.0644,0f000001,0*9acc447f\n\t", "INSPVAXA,USB3,0,46.0,FINESTEERING,2107,283743.800,02000000,471d,15824;INS_ALIGNMENT_COMPLETE,INS_RTKFIXED,37.37113371860,126.72177667415,8.0236,22.3000,-0.3426,-0.2605,-0.0024,-1.484785571,-0.050192547,211.992358658,0.4337,0.3019,0.5833,0.1132,0.0937,0.0803,0.0960,0.0999,5.0644,0f000001,0*53a396a3\n\t", "INSPVAXA,USB3,0,49.5,FINESTEERING,2107,283744.300,02000000,471d,15824;INS_ALIGNMENT_COMPLETE,INS_RTKFIXED,37.37113201879,126.72177513465,8.0232,22.3000,-0.3446,-0.2615,0.0259,-1.383371091,0.074969047,212.298273108,0.4337,0.3020,0.5833,0.1129,0.0934,0.0801,0.0960,0.0999,5.0660,0f000001,0*aa113718\n\t", "INSPVAXA,USB3,0,49.5,FINESTEERING,2107,283744.800,02000000,471d,15824;INS_ALIGNMENT_COMPLETE,INS_RTKFIXED,37.37113032635,126.72177358354,8.0234,22.3000,-0.3375,-0.2772,0.0273,-1.329281946,0.043160679,212.609113265,0.4337,0.3020,0.5833,0.1129,0.0934,0.0801,0.0960,0.0999,5.0660,0f000001,0*0ee78c5b\n\t", "INSPVAXA,USB3,0,52.0,FINESTEERING,2107,283745.300,02000000,471d,15824;INS_ALIGNMENT_COMPLETE,INS_RTKFIXED,37.37112862779,126.72177199929,8.0231,22.3000,-0.3459,-0.2782,0.0216,-1.184506207,0.212511857,212.764446314,0.4334,0.3022,0.5833,0.1126,0.0933,0.0799,0.0960,0.0999,5.0673,0f000001,0*6b47a2c0\n\t", "INSPVAXA,USB3,0,50.5,FINESTEERING,2107,283746.300,02000000,471d,15824;INS_ALIGNMENT_COMPLETE,INS_RTKFIXED,37.37112521282,126.72176875566,8.0246,22.3000,-0.3436,-0.2866,0.0107,-1.152398634,0.173487967,213.302028541,0.4332,0.3024,0.5833,0.1125,0.0932,0.0797,0.0960,0.0999,5.0684,0f000001,0*49aabec8\n\t", "INSPVAXA,USB3,0,50.5,FINESTEERING,2107,283746.800,02000000,471d,15824;INS_ALIGNMENT_COMPLETE,INS_RTKFIXED,37.37112349330,126.72176709470,8.0242,22.3000,-0.3497,-0.2797,0.0191,-1.314916766,0.110853537,213.600359109,0.4332,0.3024,0.5833,0.1125,0.0932,0.0797,0.0960,0.0999,5.0684,0f000001,0*7436a872\n\t", "INSPVAXA,USB3,0,49.0,FINESTEERING,2107,283747.300,02000000,471d,15824;INS_ALIGNMENT_COMPLETE,INS_RTKFIXED,37.37112180863,126.72176542630,8.0244,22.3000,-0.3486,-0.2973,0.0020,-1.259459400,-0.205839817,213.873121305,0.4330,0.3028,0.5834,0.1123,0.0929,0.0795,0.0961,0.0999,5.0687,0f000001,0*73ffb7ee\n\t", "INSPVAXA,USB3,0,49.0,FINESTEERING,2107,283747.800,02000000,471d,15824;INS_ALIGNMENT_COMPLETE,INS_RTKFIXED,37.37112013539,126.72176372884,8.0242,22.3000,-0.3447,-0.2936,0.0201,-1.219688710,-0.227511135,214.058949387,0.4330,0.3028,0.5834,0.1123,0.0929,0.0795,0.0961,0.0999,5.0687,0f000001,0*4b57b427\n\t", "INSPVAXA,USB3,0,51.0,FINESTEERING,2107,283748.800,02000000,471d,15824;INS_ALIGNMENT_COMPLETE,INS_RTKFIXED,37.37111693523,126.72176047327,8.0217,22.3000,-0.3794,-0.3424,0.0221,-1.127145988,-0.211560747,214.369143208,0.4328,0.3022,0.5832,0.1125,0.0931,0.0797,0.0961,0.0999,5.0695,0f000001,0*f768fbb4\n\t", "INSPVAXA,USB3,0,48.0,FINESTEERING,2107,283749.300,02000000,471d,15824;INS_ALIGNMENT_COMPLETE,INS_RTKFIXED,37.37111528295,126.72175880850,8.0228,22.3000,-0.3091,-0.2843,0.0017,-1.226699576,0.077786636,214.515601245,0.4326,0.3019,0.5831,0.1128,0.0935,0.0801,0.0961,0.1000,5.0707,0f000001,0*33e38593\n\t", "INSPVAXA,USB3,0,48.0,FINESTEERING,2107,283749.800,02000000,471d,15824;INS_ALIGNMENT_COMPLETE,INS_RTKFIXED,37.37111354772,126.72175702907,8.0230,22.3000,-0.3442,-0.3142,0.0177,-1.011041502,-0.010822308,214.650851385,0.4326,0.3019,0.5831,0.1128,0.0935,0.0801,0.0961,0.1000,5.0707,0f000001,0*157ce5bb\n\t", "INSPVAXA,USB3,0,50.0,FINESTEERING,2107,283751.300,02000000,471d,15824;INS_ALIGNMENT_COMPLETE,INS_RTKFIXED,37.37110849817,126.72175192105,8.0275,22.3000,-0.3358,-0.3126,0.0172,-1.035437411,0.273015584,214.819783864,0.4328,0.3018,0.5834,0.1129,0.0936,0.0806,0.0961,0.1000,5.0732,0f000001,0*f034d66d\n\t", "INSPVAXA,USB3,0,50.0,FINESTEERING,2107,283751.800,02000000,471d,15824;INS_ALIGNMENT_COMPLETE,INS_RTKFIXED,37.37110680705,126.72175019748,8.0301,22.3000,-0.3539,-0.3161,0.0213,-1.037720149,0.378523097,214.886319407,0.4328,0.3018,0.5834,0.1129,0.0936,0.0806,0.0961,0.1000,5.0732,0f000001,0*08748abc\n\t", "INSPVAXA,USB3,0,49.5,FINESTEERING,2107,283752.300,02000000,471d,15824;INS_ALIGNMENT_COMPLETE,INS_RTKFIXED,37.37110513951,126.72174852580,8.0342,22.3000,-0.3395,-0.3054,0.0275,-1.169969735,0.177564821,214.703949877,0.4330,0.3019,0.5837,0.1127,0.0933,0.0804,0.0962,0.1001,5.0745,0f000001,0*3b22e019\n\t", "INSPVAXA,USB3,0,49.5,FINESTEERING,2107,283752.800,02000000,471d,15824;INS_ALIGNMENT_COMPLETE,INS_RTKFIXED,37.37110344707,126.72174683245,8.0372,22.3000,-0.3480,-0.3077,0.0306,-1.217859023,0.163695826,214.472427666,0.4330,0.3019,0.5837,0.1127,0.0933,0.0804,0.0962,0.1001,5.0745,0f000001,0*0f7f998b\n\t", "INSPVAXA,USB3,0,49.0,FINESTEERING,2107,283753.300,02000000,471d,15824;INS_ALIGNMENT_COMPLETE,INS_RTKFIXED,37.37110176276,126.72174513892,8.0405,22.3000,-0.3362,-0.2959,0.0055,-0.953272899,0.159929728,214.321717849,0.4329,0.3016,0.5838,0.1125,0.0931,0.0801,0.0962,0.1001,5.0760,0f000001,0*9e9621c6\n\t", "INSPVAXA,USB3,0,49.0,FINESTEERING,2107,283753.800,02000000,471d,15824;INS_ALIGNMENT_COMPLETE,INS_RTKFIXED,37.37110008196,126.72174349775,8.0442,22.3000,-0.3613,-0.3106,0.0312,-1.166829812,0.116996203,214.014548565,0.4329,0.3016,0.5838,0.1125,0.0931,0.0801,0.0962,0.1001,5.0760,0f000001,0*f55bb199\n\t", "INSPVAXA,USB3,0,50.5,FINESTEERING,2107,283754.300,02000000,471d,15824;INS_ALIGNMENT_COMPLETE,INS_RTKFIXED,37.37109836373,126.72174184574,8.0475,22.3000,-0.3327,-0.2951,0.0321,-1.340604372,0.249067491,213.619073128,0.4327,0.3010,0.5839,0.1123,0.0933,0.0799,0.0962,0.1001,5.0774,0f000001,0*1e6eecd6\n\t", "INSPVAXA,USB3,0,50.5,FINESTEERING,2107,283754.800,02000000,471d,15824;INS_ALIGNMENT_COMPLETE,INS_RTKFIXED,37.37109667964,126.72174020389,8.0524,22.3000,-0.3499,-0.2857,0.0212,-1.089589442,0.349909054,213.310894710,0.4327,0.3010,0.5839,0.1123,0.0933,0.0799,0.0962,0.1001,5.0774,0f000001,0*4cfde7b0\n\t", "INSPVAXA,USB3,0,50.0,FINESTEERING,2107,283755.300,02000000,471d,15824;INS_ALIGNMENT_COMPLETE,INS_RTKFIXED,37.37109494631,126.72173857933,8.0558,22.3000,-0.3482,-0.3112,0.0327,-1.123456133,0.254250073,212.973630812,0.4328,0.3002,0.5840,0.1125,0.0933,0.0800,0.0962,0.1002,5.0783,0f000001,0*6370c8f7\n\t", "INSPVAXA,USB3,0,50.0,FINESTEERING,2107,283755.800,02000000,471d,15824;INS_ALIGNMENT_COMPLETE,INS_RTKFIXED,37.37109323993,126.72173698484,8.0607,22.3000,-0.3643,-0.2927,0.0186,-1.115855413,0.320489035,212.665195189,0.4328,0.3002,0.5840,0.1125,0.0933,0.0800,0.0962,0.1002,5.0783,0f000001,0*79f1de9b\n\t", "INSPVAXA,USB3,0,49.0,FINESTEERING,2107,283756.300,02000000,471d,15824;INS_ALIGNMENT_COMPLETE,INS_RTKFIXED,37.37109147412,126.72173536418,8.0658,22.3000,-0.3720,-0.2998,0.0176,-0.967758336,0.009147585,212.513392073,0.4329,0.3001,0.5842,0.1131,0.0941,0.0808,0.0962,0.1002,5.0788,0f000001,0*480160b6\n\t", "INSPVAXA,USB3,0,49.0,FINESTEERING,2107,283756.800,02000000,471d,15824;INS_ALIGNMENT_COMPLETE,INS_RTKFIXED,37.37108975069,126.72173380065,8.0704,22.3000,-0.3560,-0.3018,0.0441,-0.888869342,0.191957925,212.381344702,0.4329,0.3001,0.5842,0.1131,0.0941,0.0808,0.0962,0.1002,5.0788,0f000001,0*35d96739\n\t", "INSPVAXA,USB3,0,50.5,FINESTEERING,2107,283757.300,02000000,471d,15824;INS_ALIGNMENT_COMPLETE,INS_RTKFIXED,37.37108800138,126.72173224082,8.0747,22.3000,-0.3610,-0.2896,0.0115,-0.827433156,0.184771072,212.230918209,0.4331,0.3002,0.5847,0.1138,0.0947,0.0820,0.0961,0.1002,5.0788,0f000001,0*487ee94f\n\t", "INSPVAXA,USB3,0,50.5,FINESTEERING,2107,283757.800,02000000,471d,15824;INS_ALIGNMENT_COMPLETE,INS_RTKFIXED,37.37108628681,126.72173070436,8.0804,22.3000,-0.3571,-0.2959,0.0231,-0.782297314,0.234364659,212.024110500,0.4331,0.3002,0.5847,0.1138,0.0947,0.0820,0.0961,0.1002,5.0788,0f000001,0*d45b12f8\n\t", "INSPVAXA,USB3,0,48.5,FINESTEERING,2107,283758.300,02000000,471d,15824;INS_ALIGNMENT_COMPLETE,INS_RTKFIXED,37.37108452216,126.72172915072,8.0875,22.3000,-0.3471,-0.2721,0.0431,-0.667161405,0.478660686,212.038204919,0.4334,0.3007,0.5852,0.1141,0.0949,0.0828,0.0961,0.1002,5.0790,0f000001,0*96971f51\n\t", "INSPVAXA,USB3,0,48.5,FINESTEERING,2107,283758.800,02000000,471d,15824;INS_ALIGNMENT_COMPLETE,INS_RTKFIXED,37.37108279307,126.72172764103,8.0915,22.3000,-0.3762,-0.2924,0.0247,-0.558954729,0.708405130,211.994899529,0.4334,0.3007,0.5852,0.1141,0.0949,0.0828,0.0961,0.1002,5.0790,0f000001,0*cea2d680\n\t", "INSPVAXA,USB3,0,49.0,FINESTEERING,2107,283759.300,02000000,471d,15824;INS_ALIGNMENT_COMPLETE,INS_RTKFIXED,37.37108105868,126.72172613061,8.0959,22.3000,-0.3577,-0.2867,0.0280,-0.582378348,0.657248955,212.009317434,0.4336,0.3012,0.5858,0.1140,0.0947,0.0830,0.0962,0.1003,5.0797,0f000001,0*cc7fd0eb\n\t", "INSPVAXA,USB3,0,49.0,FINESTEERING,2107,283759.800,02000000,471d,15824;INS_ALIGNMENT_COMPLETE,INS_RTKFIXED,37.37107931872,126.72172458410,8.1011,22.3000,-0.3599,-0.2848,0.0379,-0.459271249,0.431724641,212.075547686,0.4336,0.3012,0.5858,0.1140,0.0947,0.0830,0.0962,0.1003,5.0797,0f000001,0*b3831dc9\n\t", "INSPVAXA,USB3,0,49.0,FINESTEERING,2107,283760.300,02000000,471d,15824;INS_ALIGNMENT_COMPLETE,INS_RTKFIXED,37.37107757487,126.72172306983,8.1066,22.3000,-0.3662,-0.2801,0.0079,-0.623221926,0.408229344,212.074392228,0.4338,0.3017,0.5866,0.1138,0.0944,0.0831,0.0962,0.1003,5.0809,0f000001,0*d3997e6b\n\t", "INSPVAXA,USB3,0,49.0,FINESTEERING,2107,283760.800,02000000,471d,15824;INS_ALIGNMENT_COMPLETE,INS_RTKFIXED,37.37107585658,126.72172154929,8.1105,22.3000,-0.3559,-0.2976,0.0252,-0.619300370,0.317089157,212.125818977,0.4338,0.3017,0.5866,0.1138,0.0944,0.0831,0.0962,0.1003,5.0809,0f000001,0*2578c1d0\n\t", "INSPVAXA,USB3,0,47.5,FINESTEERING,2107,283761.300,02000000,471d,15824;INS_ALIGNMENT_COMPLETE,INS_RTKFIXED,37.37107412615,126.72172002171,8.1136,22.3000,-0.3598,-0.2783,0.0314,-0.587667385,0.123936522,212.281601914,0.4339,0.3017,0.5874,0.1136,0.0941,0.0830,
